vi "Get Current Position.vi"(8 "error in":errorcluster, 11 "Axis in":refnum<class "Axis.lvclass">) -> (0 "error out":errorcluster, 2 "Current Position":dbl, 3 "Axis out":refnum<class "Axis.lvclass">)   [LabVIEW 2018, in "Axis.lvlib" / "Axis.lvclass"]
uses:
  Axis.lvclass
  Custom Controls/Command.ctl
  Axis.lvclass/Axis.ctl
  Axis.lvlib
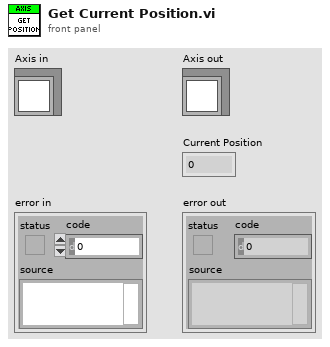
[diagram p1: front panel]
types:
  T1 = typedef "Axis.lvlib/Command.ctl" = enum16{"None", "Home", "Renumber", "Move Absolute", "Move Relative", "Stop", "Set Run Speed", "Set Acceleration", "Set Run Current", "Set Home Offset", "Set Home Speed", "Query Current Position", "Load Defaults", "Query Status", "Lock Controls", "Unlock Controls", "Set Jog Step Size", "Set Jog Acceleration", "Set Jog Speed", "Query Homed Status", "Query Moving Status", "Reset", "Set Max Position", "Set Min Position"}
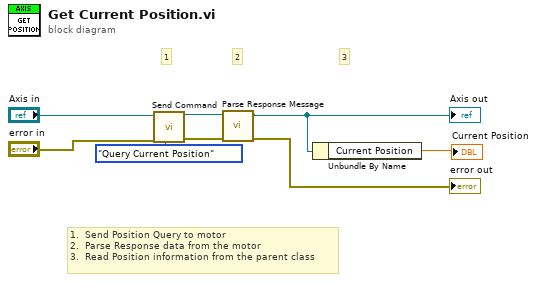
[diagram p0: block diagram]
diagram:
  # "1.  Send Position Query to motor\n2.  Parse Response data from the motor\n3.  Read Position information from the parent class"
  # "3"
  # "2"
  # "1"
  n1 = call-dynamic "Send Command.vi"("Command"=Command."Query Current Position", "error in"="error in", "Axis in"="Axis in") -> ("error out"=w3:errorcluster, "Axis out"=w4:refnum<class "Axis.lvclass">)  [unwired: 7 in]
  n2 = call-dynamic "Parse Response Message.vi"("error in"=w3, "Axis in"=w4) -> ("error out"=→"error out":errorcluster, "Axis out"=w2:refnum<class "Axis.lvclass">)  [unwired: 8 in]
  "Axis out" <- w2
  n3 = Unbundle By Name(w2) -> ("Current Position"=→"Current Position":dbl)
